vi "Ventilo.vi"(0 "Boolean":bool) -> ()   [LabVIEW 2022 SP3]
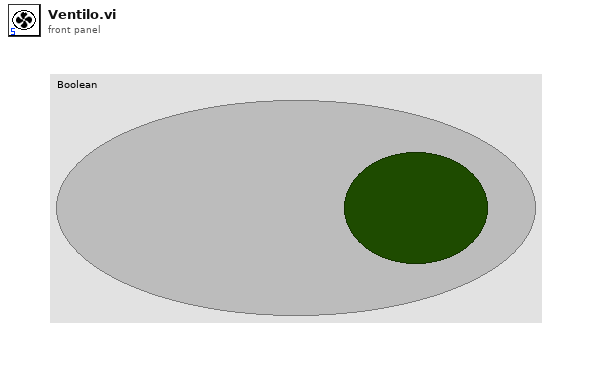
[diagram p1: front panel]
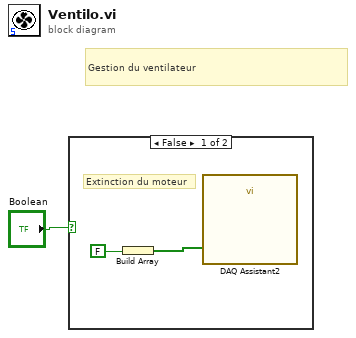
[diagram p0: block diagram]
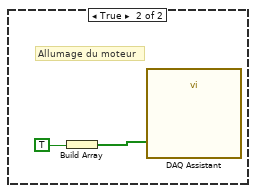
[diagram p2: hidden frame]
diagram:
  # "Gestion du ventilateur"
  n1 = case shown="False" "Boolean" {
    frame False {
      # "Extinction du moteur"
      n2 = Build Array(FALSE) -> (w3:bool[])
      n3 = call "DAQ Assistant2"("data"=w3) -> ()  [unwired: 17 in, 2 out]
    }
    frame True {
      # "Allumage du moteur"
      n4 = Build Array(TRUE) -> (w5:bool[])
      n5 = call "DAQ Assistant"("data"=w5) -> ()  [unwired: 17 in, 2 out]
    }
  }
